vi "Configure Power Line Frequency [PLF].vi"(8 "error in (no error)":errorcluster, 10 "power line frequency (60.0 Hz)":dbl=60.0 format="%^.2e", 11 "CS++DMM in":refnum<class "CS++DMM.lvclass">) -> (0 "error out":errorcluster, 3 "CS++DMM out":refnum<class "CS++DMM.lvclass">)   [LabVIEW 2015, in "CS++DMM.lvlib" / "CS++DMM.lvclass"]
doc: "This VI configures the power line frequency of the DMM.\n\nNote:\n\n(1) This VI is part of the IviDmmPowerLineFrequency [PLF] extension group."
uses:
  CS++DMM.lvclass
  CSPP_Core/Classes/CS++ProcessVariables/ProcessVariable/PV.lvclass
  PV-Enum.ctl
  CSPP_Core/Classes/CS++ProcessVariables/ProcessVariable/PV.lvclass/PV.ctl
  CS++DMM.lvclass/CS++DMM.ctl
  CSPP_Core/Classes/CS++ProcessVariables/ProcessVariable/Write Data.vi
  CSPP_Core/Classes/CS++ProcessVariables/ProcessVariable/Write Timestamp.vi
  CSPP_Core/Classes/CS++ProcessVariables/ProcessVariable/Write Quality.vi
  CSPP_Core/Classes/CS++ProcessVariables/ProcessVariable/Write status.vi
  CSPP_Core/Classes/CS++ProcessVariables/PVConnection/PVConnection.lvclass
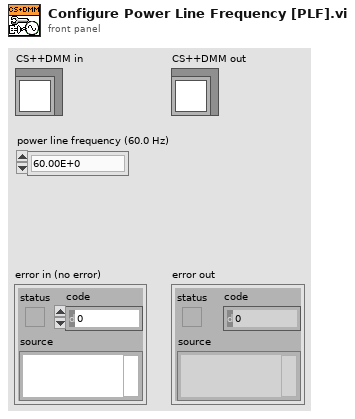
[diagram p1: front panel]
types:
  T1 = typedef "CS++DMM.lvlib/CS++DMM.lvclass/PV-Enum.ctl" = enum16{"AbsoluteResolution", "ACMaxFrequency", "ACMinFrequency", "ActualRange", "Alpha", "ApertureTime", "FixedReferenceJunction", "FrequencyVoltageRange", "PowerLineFrequency", "Range", "Reading", "Resistance", "SampleInterval", "TriggerDelay", "ApertureTimeUnit", "AutoZeroMode", "MeasCompleteDestination", "MeasurementFunction", "ReferenceJunctionType", "SampleCount", "SampleTrigger", "ThermocoupleType", "TranducerType", "TriggerCount", "TriggerSlope", "TriggerSource", "MPReading", "IsOverRange"}
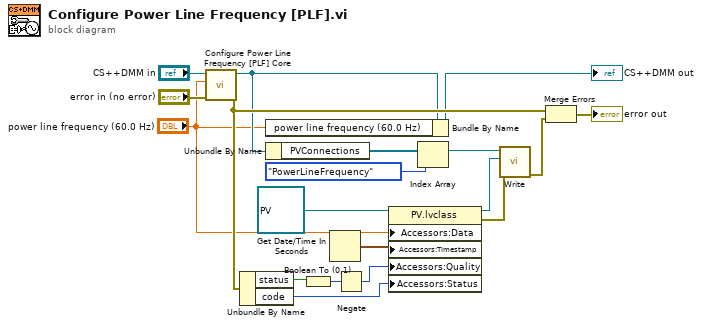
[diagram p0: block diagram]
diagram:
  n1 = call-dynamic "Configure Power Line Frequency [PLF] Core.vi"("error in (no error)"="error in (no error)", "power line frequency (60.0 Hz)"="power line frequency (60.0 Hz)", "CS++DMM in"="CS++DMM in") -> ("error out"=w7:errorcluster, "CS++DMM out"=w5:refnum<class "CS++DMM.lvclass">)  [unwired: 7 in]
  n2 = Unbundle By Name(w7) -> ("status"=w18:bool, "code"=w15:i32)
  n3 = Bundle By Name(cluster=w5, "power line frequency (60.0 Hz)"="power line frequency (60.0 Hz)") -> (→"CS++DMM out":refnum<class "CS++DMM.lvclass">)
  n4 = Unbundle By Name(w5) -> ("PVConnections"=w11:refnum<class "PVConnection.lvclass">[])
  n5 = Boolean To (0,1)(Boolean=w18) -> (0, 1=w17:i16)
  n6 = Get Date/Time In Seconds() -> (seconds since 1Jan1904=w14:timestamp)
  n7 = Negate(x=w17) -> (-x=w16:i16)
  n8 = property class="PV.lvclass"(reference=refnum<class "PV.lvclass"> refnum ("CS++ProcessVariables.lvlib:PV.lvclass"), "Accessors:Data"="power line frequency (60.0 Hz)", "Accessors:Timestamp"=w14, "Accessors:Quality"=w16, "Accessors:Status"=w15) -> (reference out=w12:refnum<class "PV.lvclass">, error out=w13:errorcluster)  [unwired: 1 in]
  n9 = Index Array(array=w11, index=PV-Enum."PowerLineFrequency" ("PV-Enum")) -> (element=w2:refnum<class "PVConnection.lvclass">)
  n10 = call "Write.vi"("error in (no error)"=w13, "PV"=w12, "PVConnection in"=w2) -> ("error out"=w10:errorcluster)  [unwired: 7 in, 1 out]
  n11 = Merge Errors(w7, w10) -> (→"error out":errorcluster)
